vi "Ophir Extract.vi"(1 "String":string="53, 42, 37") -> (0 "Single Precision Array":sgl[](array[numeric]) format="%.2f")   [LabVIEW 2017]
panel:
  # "This VI takes a string containing multiple numbers and\nextracts those numbers into an array.  See the Get Info\ndialog box for more information."
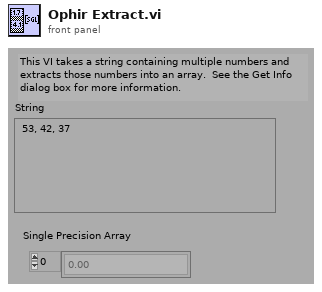
[diagram p1: front panel]
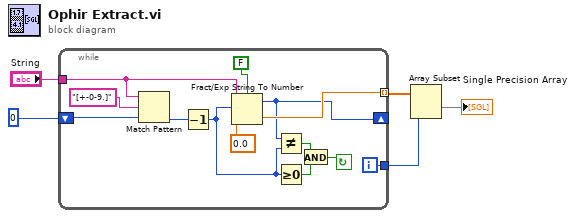
[diagram p0: block diagram]
diagram:
  n1 = while {
    tunnel: "String" -> [w12]
    tunnel: [w13] -> w3
    tunnel: [w14] -> w4 mode=indexing
    shift-left: 0 -> [w17]
    shift-right: [w8] -> _
    i -> [w13]
    stop <- w9 continue-if-true
    n2 = Match Pattern(string=w12, regular expression="[+-0-9.]", offset (0)=w17) -> (offset past match=w16:i32)  [unwired: 3 out]
    n3 = Decrement(x=w16) -> (x-1=w7:i32)
    n4 = Fract/Exp String To Number(use system decimal point (T)=FALSE, string=w12, offset=w7, default (0 dbl)=sgl 0.0) -> (offset past number=w8:i32, number=w14:sgl)
    n5 = Not Equal?(x=w8, y=w7) -> (x != y?=w11:bool)
    n6 = Greater Or Equal To 0?(x=w7) -> (x >= 0?=w10:bool)
    n7 = And(x=w11, y=w10) -> (x .and. y?=w9:bool)
  }
  n8 = Array Subset(array=w4, length=w3) -> (→"Single Precision Array":sgl[])  [unwired: 1 in]
